vi "Instantiate.vi"(1 "vi ref":refnum<vi>) -> (0 "vi ref":refnum<vi>)   [LabVIEW 2017, in "Stream-t'WPI_EncoderType.ctl'.lvlib"]
doc: "Creates and initializes the data structure that supports the channel at run time."
uses:
  <extravilib>/ChannelInstances/Stream-t'WPI_EncoderType.ctl'.lvlib
  <extravilib>/ChannelInstances/Stream-t'WPI_EncoderType.ctl'/ChannelOp.ctl
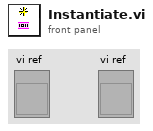
[diagram p1: front panel]
types:
  T1 = typedef "Stream-t'WPI_EncoderType.ctl'.lvlib/ChannelOp.ctl" = enum16{"init", "write", "read", "probe"}
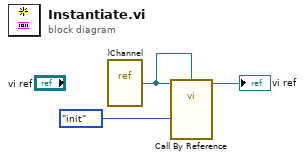
[diagram p0: block diagram]
diagram:
  n1 = vi-ref <extravilib>:")Channel.vi"() -> (w1:refnum<vi>)
  n2 = call-by-ref "?"(reference=w1, "This VI"=w1, "channelOp"=ChannelOp."init") -> (reference out=→"vi ref":refnum<vi>)  [unwired: 7 in, 9 out]
